vi "SN_TCP.vi"(7 "TServer/FClient":bool, 8 "error in (no error)":errorcluster, 9 "UseRepQ":bool, 10 "index":i32, 11 "RobotConnect":cluster{"IP":string, "Port":u16}) -> (0 "error out":errorcluster, 3 "Exit":bool)   [LabVIEW 2019]
uses:
  LLB/Message/Ctrl/MsgDataInput.ctl
  LLB/Message/Ctrl/MsgPageSelect.ctl
  LLB/Message/Ctrl/LogType.ctl
  LLB/Message/MsgShowAndLog.lvlib
  LLB/Commonly VI.lvlib
panel:
  out "RepQ":refnum<queue>
  out "Connect":refnum<vi>
  out "SN_ReplyRef":refnum<vi>
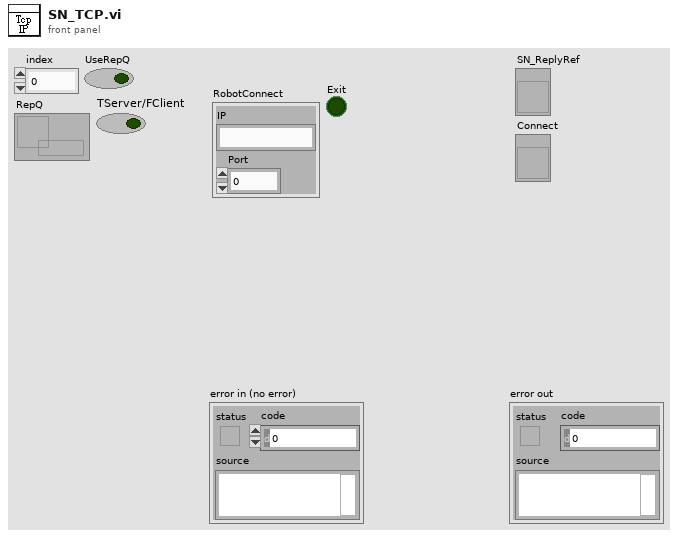
[diagram p1: front panel]
types:
  T1 = typedef "MsgDataInput.ctl" = cluster{"MsgPageSelect":T2, "LogType":T3, "Msg":string, "Time":string}
  T2 = typedef "MsgShowAndLog.lvlib/MsgPageSelect.ctl" = enum16{"System", "Comm", "IO", "Action", "Alarm"}
  T3 = typedef "MsgShowAndLog.lvlib/LogType.ctl" = enum16{"Auto", "Manual", "Handshake", "Error"}
  T4 = enum16{"Standard", "Buffered", "CRLF", "Immediate"}
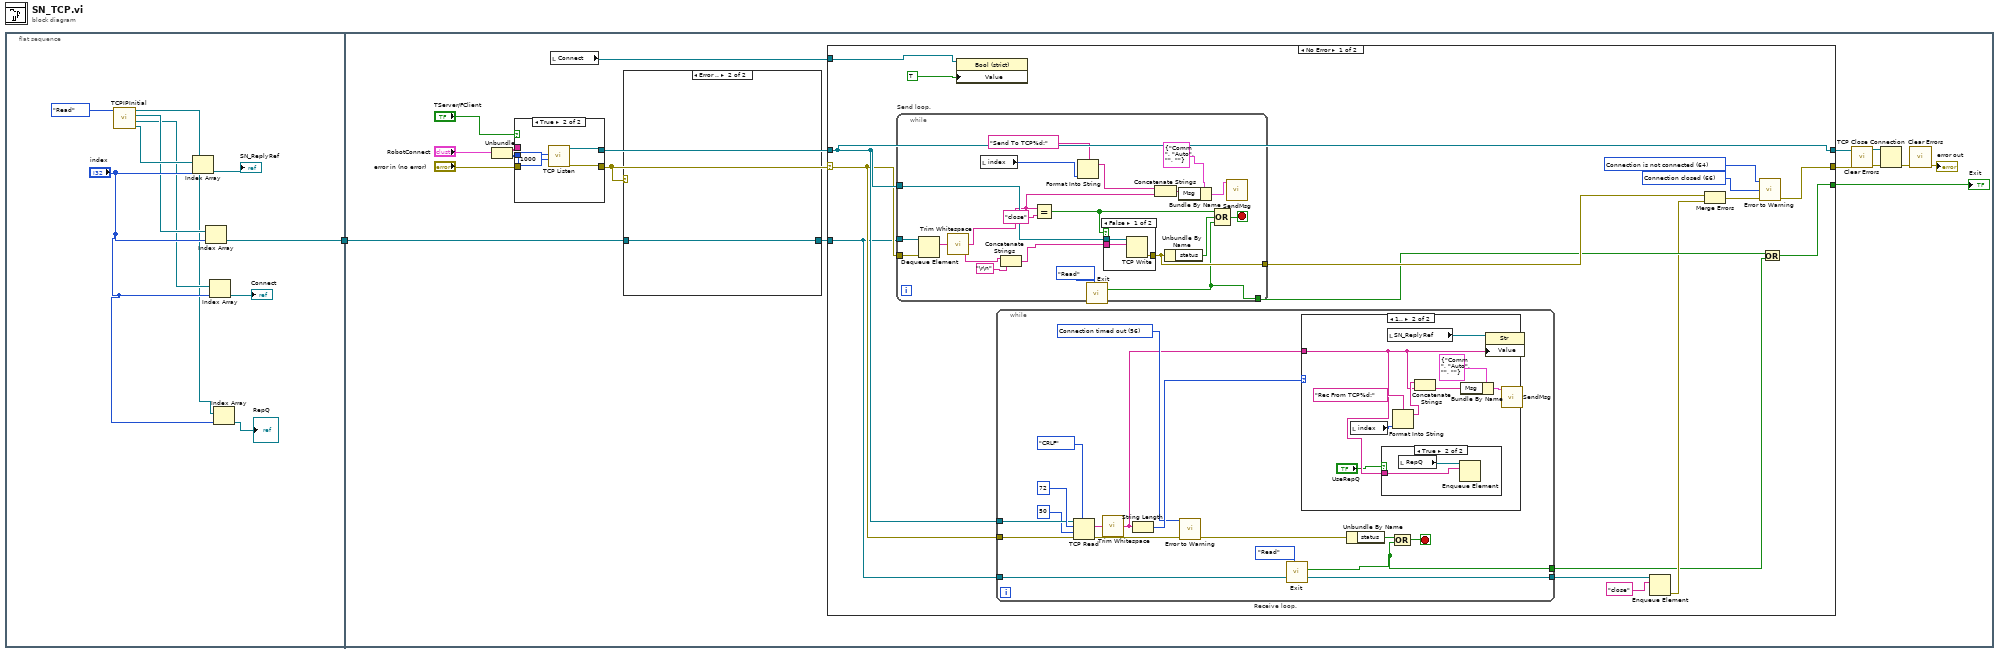
[diagram p0: block diagram]
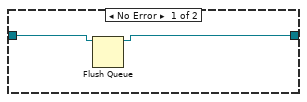
[diagram p2: hidden frame]
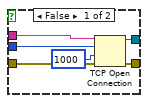
[diagram p3: hidden frame]
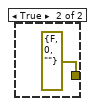
[diagram p4: hidden frame]
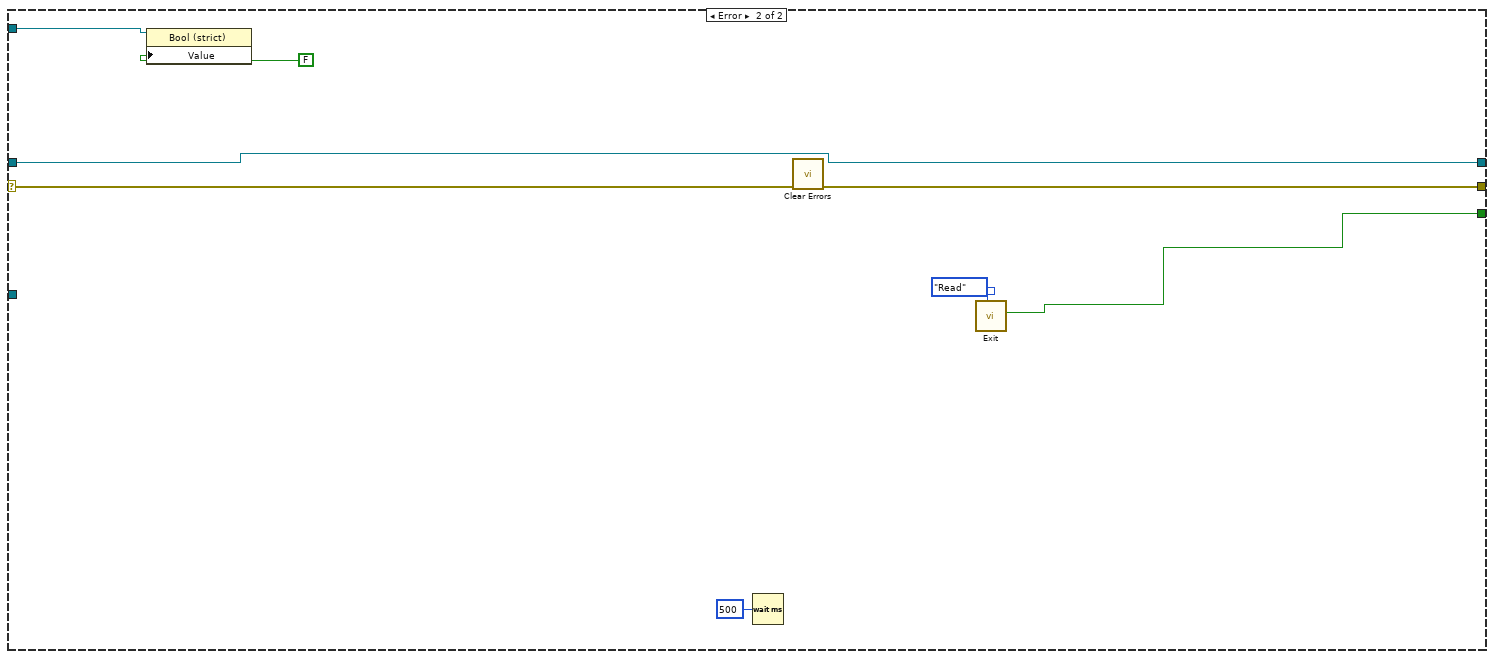
[diagram p7: hidden frame]
diagram:
  n1 = flat-sequence {
    tunnel: [w10] -> w1
    tunnel: w1 -> [w13]
    frame #0 {
      n2 = call "TCPIPInitial.vi"("Enum"=enum16{"initial", "Read", "release"}."Read") -> ("SN_ReplyRef"=w5:refnum<vi>[], "Connect"=w3:refnum<vi>[], "Sn_cmdQ"=w4:refnum<queue>[], "SN_Reply"=w2:refnum<queue>[])  [unwired: 7 in]
      n3 = Index Array(array=w5, index="index") -> (element=→"SN_ReplyRef":refnum<vi>)
      n4 = Index Array(array=w4, index="index") -> (element=w10:refnum<queue>)
      n5 = Index Array(array=w3, index="index") -> (element=→"Connect":refnum<vi>)
      n6 = Index Array(array=w2, index="index") -> (element=→"RepQ":refnum<queue>)
    }
    frame #1 {
      n7 = Unbundle("RobotConnect") -> ("IP"=w15:string, "Port"=w16:u16)
      n8 = case shown="True" "TServer/FClient" {
        tunnel: "error in (no error)" -> [w36 _]
        tunnel: [w35 w38] -> w14
        tunnel: [w34 w39] -> w25
        tunnel: w16 -> [w32 w40]
        tunnel: w15 -> [w31 _]
        frame False {
          n9 = TCP Open Connection(address=w31, remote port or service name=w32, timeout ms (60000)=1000, error in (no error)=w36) -> (connection ID=w34:refnum<k5>, error out=w35:errorcluster)  [unwired: 1 in]
        }
        frame True {
          n10 = call <vilib>:"TCP Listen.vi"("timeout ms (wait forever: -1)"=1000, "port"=w40) -> ("error out"=w38:errorcluster, "connection ID"=w39:refnum<k5>)  [unwired: 5 in, 3 out]
        }
      }
      n11 = local read "Connect"() -> (w20:refnum<vi>)
      n12 = case shown="Error .." w14 {
        tunnel: w13 -> [w29 w30]
        tunnel: [w28 w30] -> w12
        frame No Error {
          n13 = Flush Queue(queue=w29) -> (queue out=w28:refnum<queue>)  [unwired: 1 in, 2 out]
        }
        frame Error {
        }
      }
      n14 = case shown="No Error" w14 {
        selector: w14 -> [w45 w114]
        tunnel: [w51 w113] -> w23
        tunnel: w25 -> [w56 w115]
        tunnel: [w56 w115] -> w24
        tunnel: [w50 w108] -> w21
        tunnel: w12 -> [w44 _]
        tunnel: w20 -> [w42 w112]
        frame No Error {
          w52 = 66 items=["No Error", "Argument Error", "Memory Full", "Out of Zone", "End of File", "File Already Open", "Generic File IO Error", "File Not Found", "File Permission Error", "Disk Full", "Duplicate Path", "Too Many Files Open", "Not Enabled", "Resource File Not Found", "Cannot Add Resource", "Resource Not Found", "Image Not Found", "Image Memory Error", "Pen Does Not Exist", "Config Bad Type", "Config Token Not Found", "Config Parse Error", "Config Memory Error", "Bad External Code Format", "Bad External Code Offset", "External Code Not Present", "Null Window", "Destroy Window Mixup", "Null Menu", "Print Aborted", "Bad Print Record", "Print Driver Error", "Windows Error During Print", "Memory Error During Print", "Print Dialog Error", "Generic Print Error", "Invalid Device Refnum", "Device Not Found", "Device Parameter Error", "Device Unit Error", "Can't Open Device", "Device Call Aborted", "Generic Error", "Cancelled By User", "Object ID Too Low", "Object ID Too High", "Object Not In Heap", "Unknown Heap", "Bad DefProc ID", "DefProc Not In Table", "Message Out Of Range", "Null Method", "Unknown Message", "Manager Call Not Supported", "Bad address", "Connection In progress", "Connection timed out", "Connection is already in progress", "Network attribute not supported", "Network error", "Address in use", "System out of memory", "Connection aborted", "Connection refused", "Connection is not connected", "Connection is already connected", "Connection closed", "Initialize error (interapplication manager)", "Bad occurrence", "Wait on unbound occurrence handler", "Occurrence queue overflow", "Bad path", "Semaphore not signaled", "Unrecognized type (interapplication manager)"] ("3rd Error to Convert")
          w53 = 64 items=["No Error", "Argument Error", "Memory Full", "Out of Zone", "End of File", "File Already Open", "Generic File IO Error", "File Not Found", "File Permission Error", "Disk Full", "Duplicate Path", "Too Many Files Open", "Not Enabled", "Resource File Not Found", "Cannot Add Resource", "Resource Not Found", "Image Not Found", "Image Memory Error", "Pen Does Not Exist", "Config Bad Type", "Config Token Not Found", "Config Parse Error", "Config Memory Error", "Bad External Code Format", "Bad External Code Offset", "External Code Not Present", "Null Window", "Destroy Window Mixup", "Null Menu", "Print Aborted", "Bad Print Record", "Print Driver Error", "Windows Error During Print", "Memory Error During Print", "Print Dialog Error", "Generic Print Error", "Invalid Device Refnum", "Device Not Found", "Device Parameter Error", "Device Unit Error", "Can't Open Device", "Device Call Aborted", "Generic Error", "Cancelled By User", "Object ID Too Low", "Object ID Too High", "Object Not In Heap", "Unknown Heap", "Bad DefProc ID", "DefProc Not In Table", "Message Out Of Range", "Null Method", "Unknown Message", "Manager Call Not Supported", "Bad address", "Connection In progress", "Connection timed out", "Connection is already in progress", "Network attribute not supported", "Network error", "Address in use", "System out of memory", "Connection aborted", "Connection refused", "Connection is not connected", "Connection is already connected", "Connection closed", "Initialize error (interapplication manager)", "Bad occurrence", "Wait on unbound occurrence handler", "Occurrence queue overflow", "Bad path", "Semaphore not signaled", "Unrecognized type (interapplication manager)"] ("1st Error to Convert")
          n15 = while "Send loop." {
            tunnel: w56 -> [w76]
            tunnel: [w75] -> w55
            tunnel: [w61] -> w49
            tunnel: w44 -> [w70]
            tunnel: w45 -> [w69]
            stop <- w74 stop-if-true
            n16 = Dequeue Element(queue=w70, error in (no error)=w69) -> (element=w72:string)  [unwired: 1 in, 3 out]
            n17 = call <vilib>:"Trim Whitespace.vi"("string"=w72) -> ("trimmed string"=w59:string)  [unwired: 1 in]
            n18 = local read "index"() -> (w65:i32)
            n19 = Concatenate Strings(w59, "\r\n") -> (w58:string)
            n20 = Equal?(x=w59, y="close") -> (x = y?=w67:bool)
            n21 = Format Into String(format string="Send To TCP%d:" ("Type"), w65) -> (resulting string=w64:string)  [unwired: 2 in, 1 out]
            n22 = call "Exit.vi"("Enum"=enum16{"Initial", "Read", "Write"}."Read") -> ("ExitOut"=w61:bool)  [unwired: 10 in]
            n23 = case shown="False" w67 {
              tunnel: w76 -> [w79 _]
              tunnel: [w78 errorcluster {"status"=FALSE, "code"=0, "source"=""} ("error out")] -> w75
              tunnel: w58 -> [w77 _]
              frame False {
                n24 = TCP Write(connection ID=w79, data in=w77) -> (error out=w78:errorcluster)  [unwired: 2 in, 2 out]
              }
              frame True {
              }
            }
            n25 = Concatenate Strings(w64, w59) -> (w68:string)
            n26 = Unbundle By Name(w75) -> ("status"=w73:bool)
            n27 = Bundle By Name(cluster=T1 {"MsgPageSelect"=enum."Comm", "LogType"=enum."Auto", "Msg"="", "Time"=""} ("DataIn"), "Msg"=w68) -> (w62:T1)
            n28 = Compound Arithmetic op=OR(w67, w73, w61) -> (w74:bool)
            n29 = call "SendMsg.vi"("DataIn"=w62) -> ()  [unwired: 10 in, 1 out]
          }
          n30 = property class="Bool (strict)"(reference=w42, "Value"=TRUE ("Robot Connect")) -> ()  [unwired: 1 in, 2 out]
          n31 = while "Receive loop." {
            tunnel: w56 -> [w94]
            tunnel: [w82] -> w43
            tunnel: w44 -> [w84]
            tunnel: [w84] -> w46
            tunnel: w45 -> [w83]
            stop <- w87 stop-if-true
            w90 = 56 items=["No Error", "Argument Error", "Memory Full", "Out of Zone", "End of File", "File Already Open", "Generic File IO Error", "File Not Found", "File Permission Error", "Disk Full", "Duplicate Path", "Too Many Files Open", "Not Enabled", "Resource File Not Found", "Cannot Add Resource", "Resource Not Found", "Image Not Found", "Image Memory Error", "Pen Does Not Exist", "Config Bad Type", "Config Token Not Found", "Config Parse Error", "Config Memory Error", "Bad External Code Format", "Bad External Code Offset", "External Code Not Present", "Null Window", "Destroy Window Mixup", "Null Menu", "Print Aborted", "Bad Print Record", "Print Driver Error", "Windows Error During Print", "Memory Error During Print", "Print Dialog Error", "Generic Print Error", "Invalid Device Refnum", "Device Not Found", "Device Parameter Error", "Device Unit Error", "Can't Open Device", "Device Call Aborted", "Generic Error", "Cancelled By User", "Object ID Too Low", "Object ID Too High", "Object Not In Heap", "Unknown Heap", "Bad DefProc ID", "DefProc Not In Table", "Message Out Of Range", "Null Method", "Unknown Message", "Manager Call Not Supported", "Bad address", "Connection In progress", "Connection timed out", "Connection is already in progress", "Network attribute not supported", "Network error", "Address in use", "System out of memory", "Connection aborted", "Connection refused", "Connection is not connected", "Connection is already connected", "Connection closed", "Initialize error (interapplication manager)", "Bad occurrence", "Wait on unbound occurrence handler", "Occurrence queue overflow", "Bad path", "Semaphore not signaled", "Unrecognized type (interapplication manager)"] ("1st Error to Convert")
            n32 = TCP Read(connection ID=w94, bytes to read=72, error in (no error)=w83, 7:T4."CRLF" ("mode (standard)"), 9:50) -> (data out=w93:string, error out=w91:errorcluster)  [unwired: 1 out]
            n33 = call <vilib>:"Trim Whitespace.vi"("string"=w93) -> ("trimmed string"=w86:string)  [unwired: 1 in]
            n34 = String Length(string=w86) -> (length=w96:i32)
            n35 = call <vilib>:"Error to Warning.vi"("1st Error to Convert"=w90, "error in"=w91) -> ("warning out"=w89:errorcluster)  [unwired: 13 in]
            n36 = call "Exit.vi"("Enum"=enum16{"Initial", "Read", "Write"}."Read") -> ("ExitOut"=w82:bool)  [unwired: 10 in]
            n37 = case shown="1.." w96 {
              tunnel: w86 -> [_ w99]
              frame ..0 {
              }
              frame 1.. {
                n38 = local read "index"() -> (w102:i32)
                n39 = case shown="True" "UseRepQ" {
                  tunnel: w99 -> [_ w106]
                  frame False {
                  }
                  frame True {
                    n40 = local read "RepQ"() -> (w107:refnum<queue>)
                    n41 = Enqueue Element(queue=w107, element=w106) -> ()  [unwired: 2 in, 3 out]
                  }
                }
                n42 = local read "SN_ReplyRef"() -> (w103:refnum<vi>)
                n43 = Format Into String(format string="Rec From TCP%d:" ("Type"), w102) -> (resulting string=w100:string)  [unwired: 2 in, 1 out]
                n44 = Concatenate Strings(w100, w99) -> (w104:string)
                n45 = Bundle By Name(cluster=T1 {"MsgPageSelect"=enum."Comm", "LogType"=enum."Auto", "Msg"="", "Time"=""} ("DataIn"), "Msg"=w104) -> (w105:T1)
                n46 = property class="Str"(reference=w103, "Value"=w99) -> ()  [unwired: 1 in, 2 out]
                n47 = call "SendMsg.vi"("DataIn"=w105) -> ()  [unwired: 10 in, 1 out]
              }
            }
            n48 = Unbundle By Name(w89) -> ("status"=w85:bool)
            n49 = Compound Arithmetic op=OR(w85, w82) -> (w87:bool)
          }
          n50 = Enqueue Element(queue=w46, element="close") -> (error out=w47:errorcluster)  [unwired: 2 in, 2 out]
          n51 = Merge Errors(w55, w47) -> (w54:errorcluster)
          n52 = call <vilib>:"Error to Warning.vi"("1st Error to Convert"=w53, "3rd Error to Convert"=w52, "error in"=w54) -> ("warning out"=w51:errorcluster)  [unwired: 12 in]
          n53 = Or(x=w49, y=w43) -> (x .or. y?=w50:bool)
        }
        frame Error {
          n54 = property class="Bool (strict)"(reference=w112, "Value"=FALSE ("Robot Connect")) -> ()  [unwired: 1 in, 2 out]
          n55 = Wait (ms)(milliseconds to wait=u32 500) -> ()  [unwired: 1 out]
          n56 = call <vilib>:"Clear Errors.vi"("error in (no error)"=w114) -> ("error out"=w113:errorcluster)  [unwired: 5 in, 1 out]
          n57 = call "Exit.vi"("Enum"=enum16{"Initial", "Read", "Write"}."Read") -> ("ExitOut"=w108:bool)  [unwired: 10 in]
        }
      }
      "Exit" <- w21
      n58 = call <vilib>:"Clear Errors.vi"("error in (no error)"=w23) -> ("error out"=w19:errorcluster)  [unwired: 5 in, 1 out]
      n59 = TCP Close Connection(connection ID=w24, error in (no error)=w19) -> (error out=w22:errorcluster)  [unwired: 1 in, 1 out]
      n60 = call <vilib>:"Clear Errors.vi"("error in (no error)"=w22) -> ("error out"=→"error out":errorcluster)  [unwired: 5 in, 1 out]
    }
  }
